vi "test.vi"() -> ()   [LabVIEW 2014]
panel:
  out "Waveform Chart":dbl(graph)
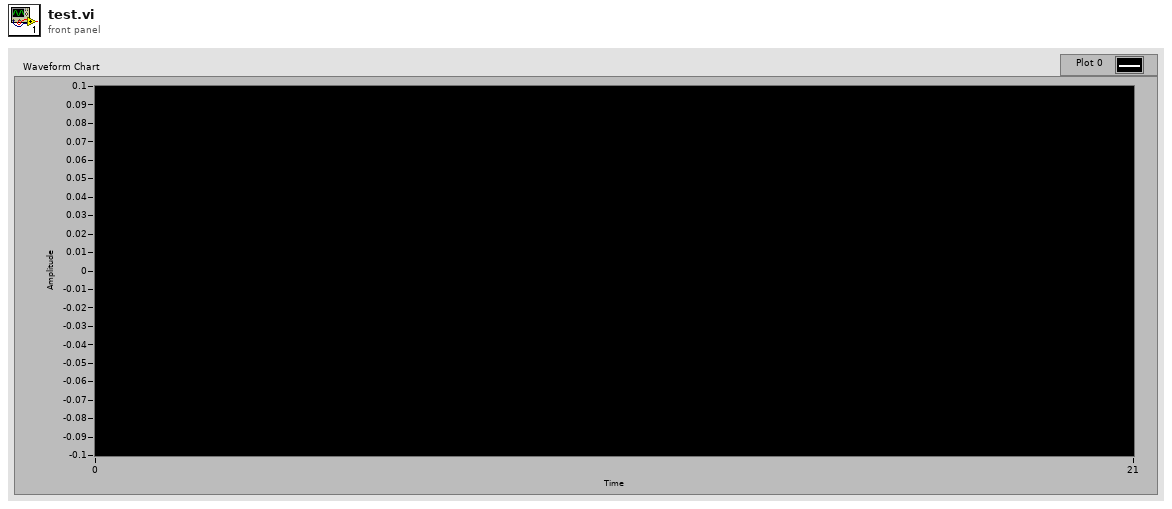
[diagram p1: front panel]
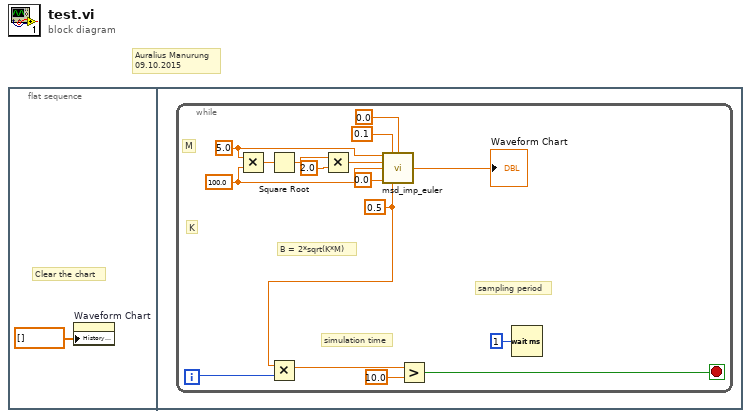
[diagram p0: block diagram]
diagram:
  # "Auralius Manurung\n09.10.2015"
  n1 = flat-sequence {
    frame #0 {
      # "Clear the chart"
      n2 = property on="Waveform Chart" class="WFChart (strict)"("History Data"=dbl[] []) -> ()  [unwired: 2 in, 2 out]
    }
    frame #1 {
      n3 = while {
        i -> [w6]
        stop <- w3 stop-if-true
        w2 = 0.5 ("h")
        w12 = 100.0 ("K")
        w16 = 5.0 ("M")
        # "simulation time"
        # "sampling period"
        # "B = 2*sqrt(K*M)"
        # "K"
        # "M"
        n4 = Multiply(x=w16, y=w12) -> (x*y=w15:dbl)
        n5 = Square Root(x=w15) -> (sqrt(x)=w14:dbl)
        n6 = Multiply(x=w2, y=w6) -> (x*y=w5:dbl)
        n7 = Multiply(x=w14, y=2.0) -> (x*y=w7:dbl)
        n8 = call "msd_imp_euler.vi"("M"=w16, "x0"=0.1, "v0"=0.0, "B"=w7, "K"=w12, "F"=0.0, "h"=w2) -> ("x1"=→"Waveform Chart":dbl)  [unwired: 8 in]
        n9 = Greater?(x=w5, y=10.0) -> (0:w3:bool)
        n10 = Wait (ms)(milliseconds to wait=u32 1) -> ()  [unwired: 1 out]
      }
    }
  }
